vi "Open Audio File Write (WAV) (Core).vi"(8 "error in (no error)":errorcluster, 9 "Codec Specific Info":T1={"Container Format"=enum."RIFF", "Data Format"=1} {"Data Format" items=["PCM"=1, "ADPCM"=2, "IEEE Float"=3]}, 10 "Audio File Info":T4={"Sample Rate (Hz)"=44100, "Channels"=2, "Bit Depth"=16}, 11 "Path":string) -> (0 "error out":errorcluster, 3 "Audio File Refnum":T5)   [LabVIEW 2020, in "G-Audio.lvlib"]
doc: "Create or replace an audio file and initialize the WAV encoder for writing."
uses:
  G-Audio.lvlib
  Controls/Audio File Info.ctl
  Controls/WAV Codec Specific Info.ctl
  Controls/WAV Container Format.ctl
  Controls/WAV Data Format.ctl
  Controls/Audio File Codec.ctl
  <vilib>/Utility/error.llb/Error Cluster From Error Code.vi
  lib/g_audio_32.dll
  Controls/Audio File Refnum.ctl
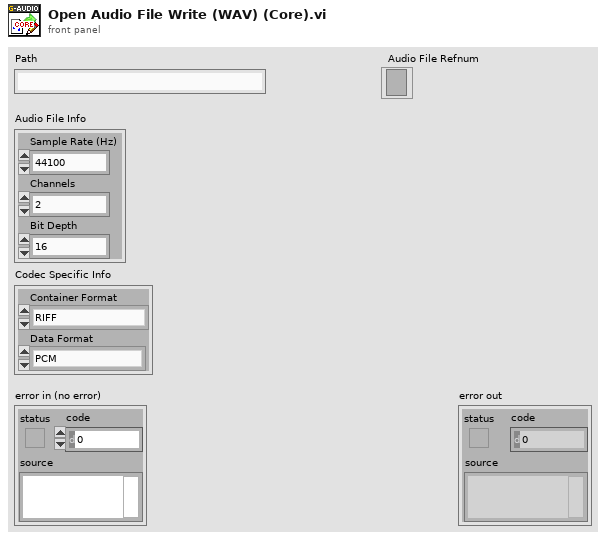
[diagram p1: front panel]
types:
  T1 = typedef "G-Audio.lvlib/WAV Codec Specific Info.ctl" = cluster{"Container Format":T2, "Data Format":T3}
  T2 = typedef "G-Audio.lvlib/WAV Container Format.ctl" = enum32{"RIFF", "Wave64"}
  T3 = typedef "G-Audio.lvlib/WAV Data Format.ctl" = u32
  T4 = typedef "G-Audio.lvlib/Audio File Info.ctl" = cluster{"Sample Rate (Hz)":u32, "Channels":u32, "Bit Depth":u32}
  T5 = typedef "G-Audio.lvlib/Audio File Refnum.ctl" = refnum<file>
  T6 = typedef "G-Audio.lvlib/Audio File Codec.ctl" = enum16{"flac", "mp3", "vorbis", "wav", "unsupported"}
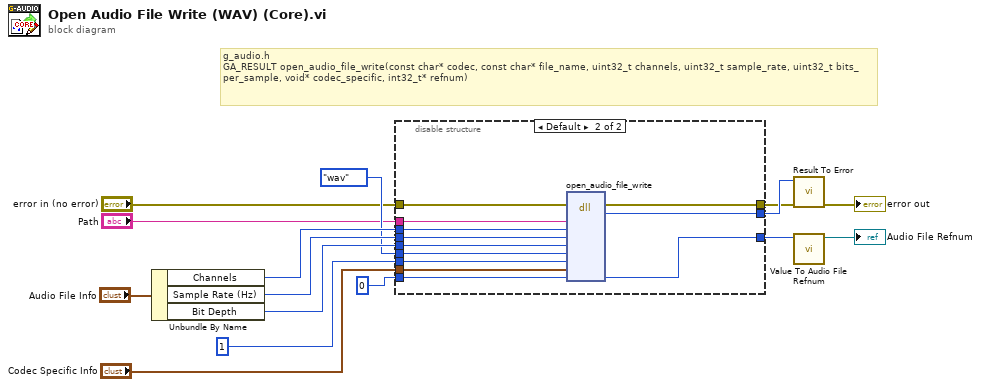
[diagram p0: block diagram]
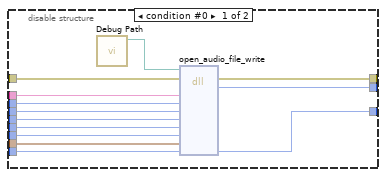
[diagram p2: hidden frame]
diagram:
  # "g_audio.h\nGA_RESULT open_audio_file_write(const char* codec, const char* file_name, uint32_t channels, uint32_t sample_rate, uint32_t bits_per_sample, void* codec_specific, int32_t* refnum)"
  n1 = Unbundle By Name("Audio File Info") -> ("Channels"=w10:u32, "Sample Rate (Hz)"=w9:u32, "Bit Depth"=w8:u32)
  n2 = disable-structure shown="Default" {
    disable-tunnel: "error in (no error)" -> [w28 w40]
    disable-tunnel: "Path" -> [w26 w38]
    disable-tunnel: [w27 w39] -> w12
    disable-tunnel: 0 ("num_samples") -> [w25 w37]
    disable-tunnel: [w24 w36] -> w1
    disable-tunnel: [w23 w35] -> w13
    disable-tunnel: w10 -> [w21 w34]
    disable-tunnel: w9 -> [w20 w33]
    disable-tunnel: w8 -> [w19 w32]
    disable-tunnel: "Codec Specific Info" -> [w18 w31]
    disable-tunnel: 1 -> [w17 w30]
    disable-tunnel: Audio_File_Codec."wav" ("Codec") -> [w16 w29]
    frame condition #0 {
      n3 = call "Debug Path.vi"() -> ("Debug Path"=w22:path)  [unwired: 11 in]
      n4 = dll-call lib="?" fn="open_audio_file_write"(path in=w22, error in=w28, "file_name"=w26, "channels"=w21, "sample_rate"=w20, "bits_per_sample"=w19, "codec"=w16, "has_specific_info"=w17, "codec_specific"=w18, "refnum"=w25) -> (error out=w27:errorcluster, "result"=w23:i32, "refnum"=w24:i32)  [unwired: 8 in, 1 out]
    }
    frame condition #1 (active) {
      n5 = dll-call lib="C:/github/dataflowg/g-audio/src/LabVIEW/G-Audio/lib/g_audio_*.*" fn="open_audio_file_write"(error in=w40, "file_name"=w38, "channels"=w34, "sample_rate"=w33, "bits_per_sample"=w32, "codec"=w29, "has_specific_info"=w30, "codec_specific"=w31, "refnum"=w37) -> (error out=w39:errorcluster, "result"=w35:i32, "refnum"=w36:i32)  [unwired: 9 in, 1 out]
    }
  }
  n6 = call "Result To Error.vi"("error in (no error)"=w12, "Result Code"=w13) -> ("error out"=→"error out":errorcluster)  [unwired: 9 in]
  n7 = call "Value To Audio File Refnum.vi"("Refnum Value"=w1) -> ("Audio File Refnum"=→"Audio File Refnum":T5)  [unwired: 10 in]
